vi "fetch_image_processor_update.vi"(8 "error in (no error)":errorcluster, 11 "DL090216Display in":refnum<class "DisplayDL090216.lvclass">) -> (0 "error out":errorcluster, 3 "DL090216Display out":refnum<class "DisplayDL090216.lvclass">)   [LabVIEW 2010, in "DisplayDL090216.lvclass"]
uses:
  DisplayDL090216.lvclass
  ImageProcessor/GenericImageProcessor/GenericImageProcessor/GenericImageProcessor.lvclass
  DisplayDL090216.lvclass/DisplayDL090216.ctl
  ImageProcessor/ImageProcessorDL090216RangeOffset/ImageProcessorDL090216RangeOffset/ImageProcessorDL090216RangeOffset.lvclass
  common/classes/ErrorController/ErrorController/class_data.vi
  common/classes/GenericComponent/GenericComponent/GenericComponent.lvclass
  common/classes/ErrorController/ErrorController/ErrorController.lvclass
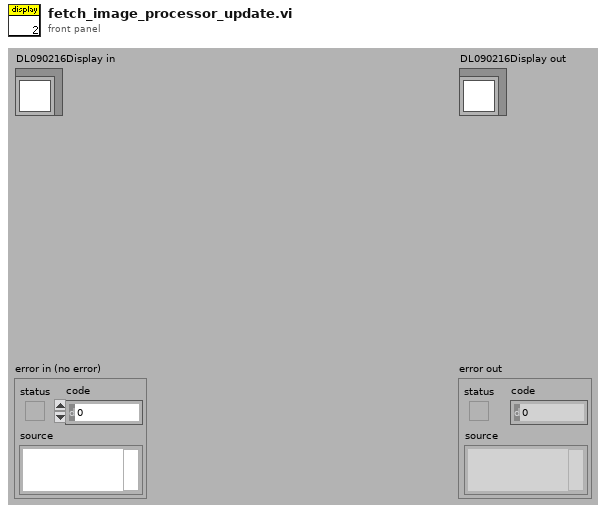
[diagram p1: front panel]
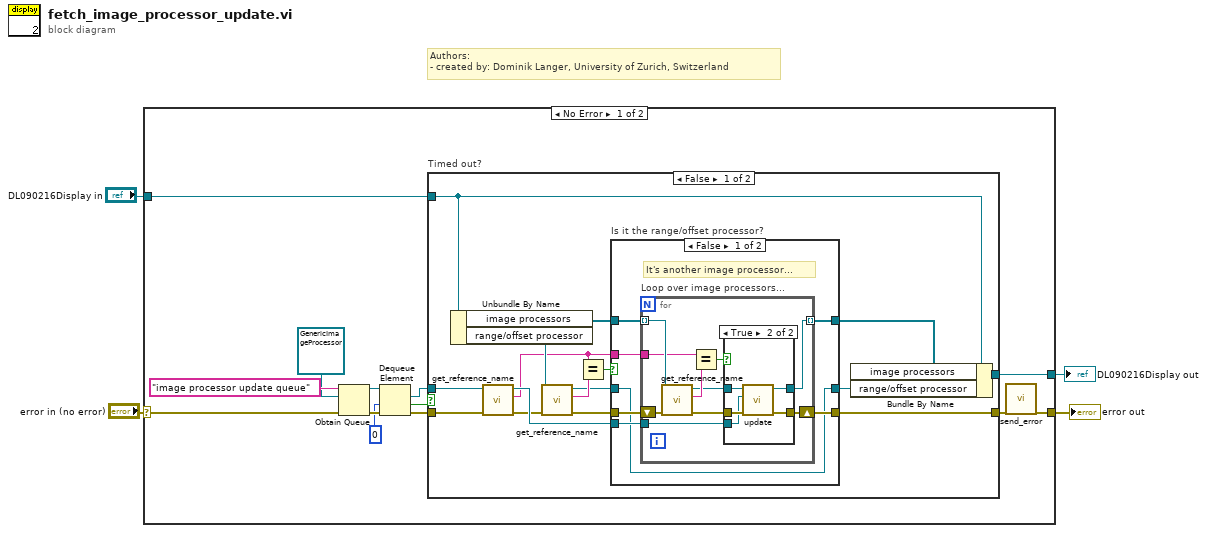
[diagram p0: block diagram]
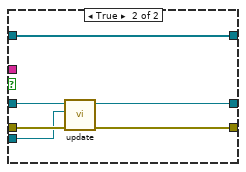
[diagram p3: hidden frame]
diagram:
  # "Authors: \n- created by: Dominik Langer, University of Zurich, Switzerland"
  n1 = case shown="No Error" "error in (no error)" {
    selector: "error in (no error)" -> [w13 w67]
    tunnel: [w6 w67] -> w3
    tunnel: [w9 w66] -> w1
    tunnel: "DL090216Display in" -> [w10 w66]
    frame No Error {
      n2 = Obtain Queue(name (unnamed)="image processor update queue", element data type=refnum<class "GenericImageProcessor.lvclass"> refnum ("GenericImageProcessor.lvclass"), error in (no error)=w13) -> (queue out=w15:refnum<queue>, error out=w14:errorcluster)  [unwired: 2 in, 1 out]
      n3 = Dequeue Element(queue=w15, timeout in ms (-1)=0, error in (no error)=w14) -> (element=w11:refnum<class "GenericImageProcessor.lvclass">, timed out?=w7:bool, error out=w12:errorcluster)  [unwired: 1 out]
      n4 = case "Timed out?" shown="False" w7 {
        tunnel: w12 -> [w33 w65]
        tunnel: [w32 w65] -> w5
        tunnel: w11 -> [w31 _]
        tunnel: w10 -> [w30 w64]
        tunnel: [w29 w64] -> w9
        frame False {
          n5 = Unbundle By Name(w30) -> ("image processors"=w24:refnum<class "GenericImageProcessor.lvclass">[], "range/offset processor"=w27:refnum<class "ImageProcessorDL090216RangeOffset.lvclass">)
          n6 = call "get_reference_name.vi"("error in (no error)"=w33, "GenericPlugin.lvclass in"=w31) -> ("error out"=w26:errorcluster, "reference name"=w23:string, "GenericPlugin.lvclass out"=w28:refnum<class "GenericImageProcessor.lvclass">)  [unwired: 7 in]
          n7 = call "get_reference_name.vi"("error in (no error)"=w26, "GenericPlugin.lvclass in"=w27) -> ("error out"=w25:errorcluster, "reference name"=w22:string, "GenericPlugin.lvclass out"=w20:refnum<class "ImageProcessorDL090216RangeOffset.lvclass">)  [unwired: 7 in]
          n8 = Equal?(x=w23, y=w22) -> (x = y?=w21:bool)
          n9 = case "Is it the range/offset processor?" shown="False" w21 {
            tunnel: [w40 w60] -> w32
            tunnel: w28 -> [w39 w61]
            tunnel: w25 -> [w38 w63]
            tunnel: w24 -> [w37 w59]
            tunnel: w23 -> [w36 _]
            tunnel: w20 -> [w34 w62]
            tunnel: [w35 w59] -> w19
            tunnel: [w34 w58] -> w18
            frame False {
              # "It's another image processor..."
              n10 = for "Loop over image processors..." {
                shift-right: [w45] -> w40
                shift-left: w38 -> [w49]
                tunnel: w37 -> [w50] mode=indexing
                tunnel: w36 -> [w48]
                tunnel: w39 -> [w42]
                tunnel: [w41] -> w35 mode=indexing
                n11 = call "get_reference_name.vi"("error in (no error)"=w49, "GenericPlugin.lvclass in"=w50) -> ("error out"=w46:errorcluster, "reference name"=w47:string, "GenericPlugin.lvclass out"=w43:refnum<class "GenericImageProcessor.lvclass">)  [unwired: 7 in]
                n12 = Equal?(x=w48, y=w47) -> (x = y?=w44:bool)
                n13 = case shown="True" w44 {
                  tunnel: w46 -> [w52 w57]
                  tunnel: [w52 w56] -> w45
                  tunnel: w43 -> [w51 w55]
                  tunnel: w42 -> [_ w54]
                  tunnel: [w51 w53] -> w41
                  frame False {
                  }
                  frame True {
                    n14 = call-dynamic "update.vi"("error in (no error)"=w57, "update"=w54, "GenericImageProcessor in"=w55) -> ("error out"=w56:errorcluster, "GenericImageProcessor out"=w53:refnum<class "GenericImageProcessor.lvclass">)  [unwired: 7 out]
                  }
                }
              }
            }
            frame True {
              n15 = call-dynamic "update.vi"("error in (no error)"=w63, "update"=w61, "DL090216RangeOffsetImageProcessor in"=w62) -> ("error out"=w60:errorcluster, "DL090216RangeOffsetImageProcessor out"=w58:refnum<class "ImageProcessorDL090216RangeOffset.lvclass">)  [unwired: 7 out]
            }
          }
          n16 = Bundle By Name(cluster=w30, "image processors"=w19, "range/offset processor"=w18) -> (w29:refnum<class "DisplayDL090216.lvclass">)
        }
        frame True {
        }
      }
      n17 = call "send_error.vi"("error in (no error)"=w5) -> ("error out"=w6:errorcluster)  [unwired: 10 in]
    }
    frame Error {
    }
  }
  "error out" <- w3
  "DL090216Display out" <- w1
